vi "Queue Last Ack.vi"(10 "Queue jettl":refnum<class "Queue jettl.lvclass">, 11 "Queue Last Ack in":refnum<class "Queue Last Ack.lvclass">) -> (3 "Queue Last Ack out":refnum<class "Queue Last Ack.lvclass">)   [LabVIEW 2021, in "jettl.lvlib" / "Queue Last Ack.lvlib" / "Queue Last Ack.lvclass"]
uses:
  Queue Last Ack.lvclass
  Queue jettl/Queue jettl.lvclass
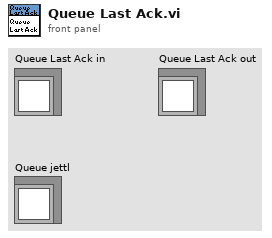
[diagram p1: front panel]
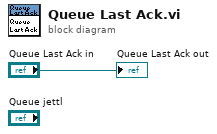
[diagram p0: block diagram]
diagram:
  "Queue Last Ack out" <- "Queue Last Ack in"
